vi "LMS151.vi"(9 "Draw Area Size":T1, 10 "stop":bool, 11 "address":string="192.168.1.7") -> (2 "Decoded Data":dbl[](array[numeric]) format="%.2f", 3 "new picture":picture)   [LabVIEW 2009]
uses:
  <vilib>/Utility/miscctls.llb/LVBoundsTypeDef.ctl
panel:
  in  "error in":errorcluster
  out "connection ID":refnum<k5>
  out "Response":string
  out "Status":string
  out "error out":errorcluster
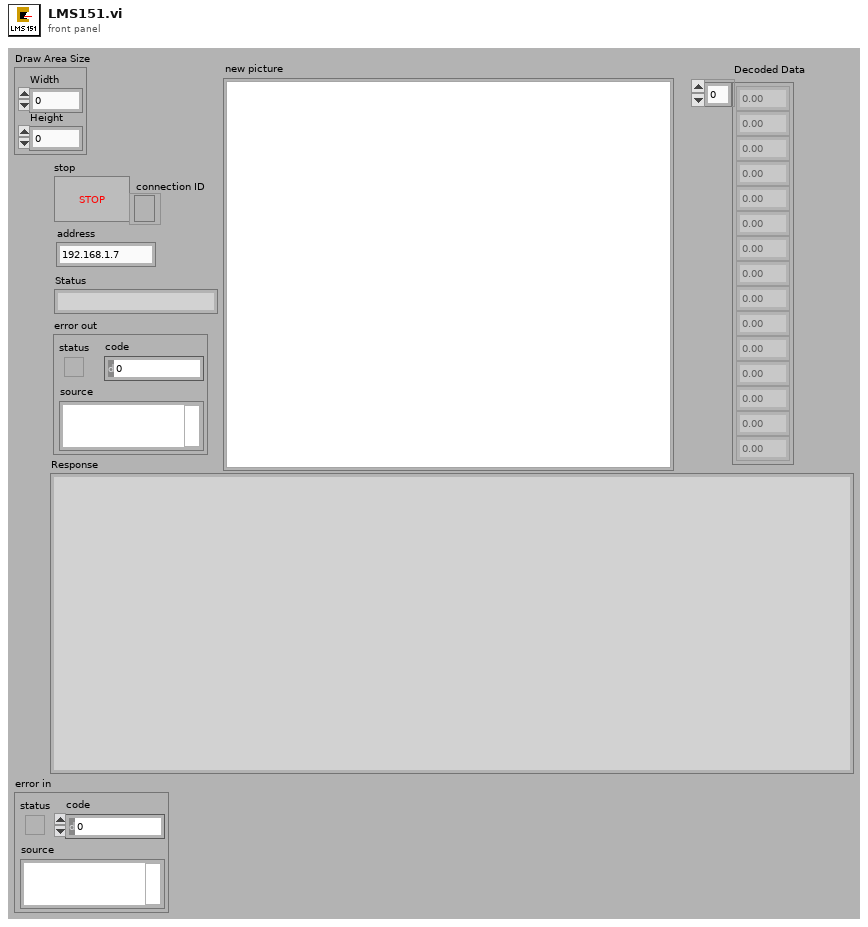
[diagram p1: front panel]
types:
  T1 = typedef "LVBoundsTypeDef.ctl" = cluster{"Width":u32, "Height":u32}
  T2 = cluster{"maximum":dbl, "minimum":dbl, "clip to min":bool, "log?(F)":bool, "grid color":u32, "plot color":u32, "fmt and prec":cluster{"format":enum8{"Decimal", "Scientific", "Engineering", "Binary", "Octal", "Hex"}, "precision":u8}, "visible section":u16}
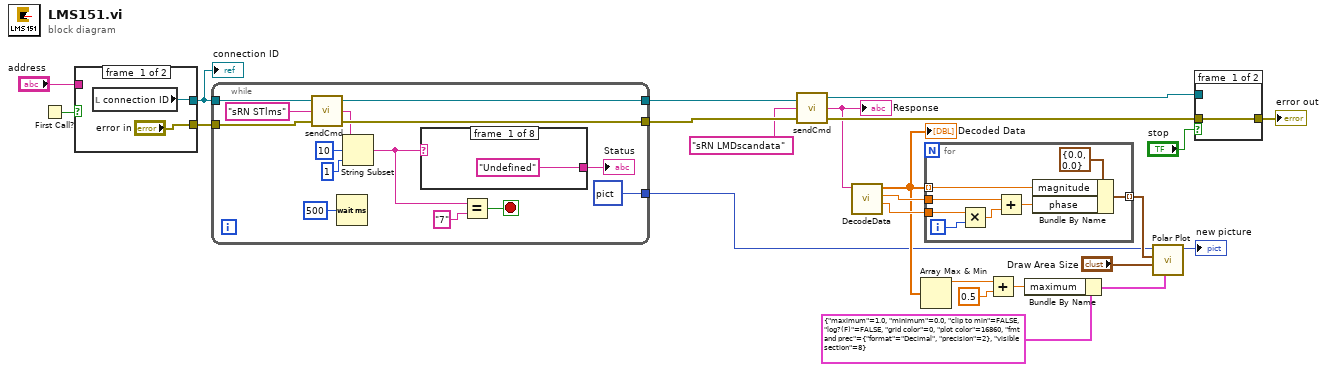
[diagram p0: block diagram]
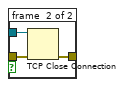
[diagram p2: hidden frame]
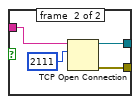
[diagram p3: hidden frame]
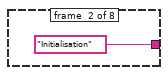
[diagram p4: hidden frame]
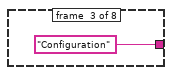
[diagram p5: hidden frame]
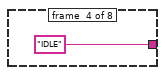
[diagram p6: hidden frame]
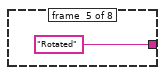
[diagram p7: hidden frame]
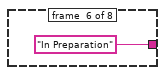
[diagram p8: hidden frame]
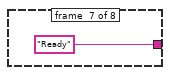
[diagram p9: hidden frame]
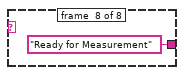
[diagram p10: hidden frame]
diagram:
  n1 = First Call?() -> (First Call?: T/F=w19:bool)
  n2 = case shown="True" w19 {
    tunnel: "address" -> [_ w29]
    tunnel: [w26 w28] -> w17
    tunnel: ["error in" w27] -> w16
    frame #0 {
      n3 = local read "connection ID"() -> (w26:refnum<k5>)
    }
    frame #1 {
      n4 = TCP Open Connection(address=w29, remote port or service name=u16 2111) -> (connection ID=w28:refnum<k5>, error out=w27:errorcluster)  [unwired: 3 in]
    }
  }
  "connection ID" <- w17
  n5 = while {
    tunnel: w17 -> [w37]
    tunnel: w16 -> [w36]
    tunnel: [w34] -> w23
    tunnel: [w35] -> w22
    tunnel: [picture data[5B] ("picture")] -> w2
    stop <- w39 stop-if-true
    n6 = call "sendCmd.vi"("error in"=w36, "Command"="sRN STlms", "connection ID"=w37) -> ("error out"=w35:errorcluster, "Response"=w32:string, "connection ID"=w34:refnum<k5>)
    n7 = Wait (ms)(milliseconds to wait=u32 500) -> ()  [unwired: 1 out]
    n8 = String Subset(string=w32, offset (0)=10, length (rest)=1 ("length (rest)")) -> (substring=w41:string)
    n9 = case shown="\"0\", Default" w41 {
      tunnel: ["Undefined" "Initialisation" "Configuration" "IDLE" "Rotated" "In Preparation" "Ready" "Ready for Measurement"] -> w42
      frame #0 {
      }
      frame #1 {
      }
      frame #2 {
      }
      frame #3 {
      }
      frame #4 {
      }
      frame #5 {
      }
      frame #6 {
      }
      frame #7 {
      }
    }
    "Status" <- w42
    n10 = Equal?(x=w41, y="7") -> (x = y?=w39:bool)
  }
  n11 = call "sendCmd.vi"("error in"=w22, "Command"="sRN LMDscandata", "connection ID"=w23) -> ("error out"=w20:errorcluster, "Response"=w14:string, "connection ID"=w21:refnum<k5>)
  "Response" <- w14
  n12 = call "DecodeData.vi"("Input Data"=w14) -> ("Angular Step Width"=w11:dbl, "Starting Angle"=w10:dbl, "Decoded Data"=w8:dbl[])  [unwired: 8 in]
  "Decoded Data" <- w8
  n13 = Array Max & Min(array=w8) -> (max value=w4:dbl)  [unwired: 3 out]
  n14 = for {
    tunnel: w8 -> [w54] mode=indexing
    tunnel: w11 -> [w56]
    tunnel: w10 -> [w55]
    tunnel: [w53] -> w9 mode=indexing
    i -> [w58]
    n15 = Multiply(x=w56, y=w58) -> (x*y=w57:dbl)
    n16 = Add(x=w55, y=w57) -> (x+y=w59:dbl)
    n17 = Bundle By Name(cluster=cluster{"magnitude":dbl, "phase":dbl} {"magnitude"=0.0, "phase"=0.0}, "magnitude"=w54, "phase"=w59) -> (w53:cluster{"magnitude":dbl, "phase":dbl})
  }
  n18 = Add(x=w4, y=0.5) -> (x+y=w5:dbl)
  n19 = Bundle By Name(cluster=T2 {"maximum"=1.0, "minimum"=0.0, "clip to min"=FALSE, "log?(F)"=FALSE, "grid color"=0, "plot color"=16860, "fmt and prec"={"format"=enum."Decimal", "precision"=2}, "visible section"=8} ("polar attributes"), "maximum"=w5) -> (w7:T2)
  n20 = call <vilib>:"Polar Plot.vi"("polar attributes"=w7, "dimensions (w,h)"="Draw Area Size", "data array [mag, phase (deg)]"=w9, "picture"=w2) -> ("new picture"=→"new picture":picture)  [unwired: 7 in]
  n21 = case shown="True" "stop" {
    tunnel: [w61 w64] -> w24
    tunnel: w21 -> [_ w63]
    tunnel: w20 -> [w61 w62]
    frame #0 {
    }
    frame #1 {
      n22 = TCP Close Connection(connection ID=w63, error in (no error)=w62) -> (error out=w64:errorcluster)  [unwired: 1 in, 1 out]
    }
  }
  "error out" <- w24
